vi "GFITS_writeFromBuffer.vi"(0 "total pixels":u32, 1 "log file":path, 2 "Database RefNum out":T1, 5 "bpp":i16=-32, 7 "buffer pointer":u32, 9 "name":string, 11 "error in (no error)":errorcluster) -> (15 "error out":errorcluster)   [LabVIEW 2016]
uses:
  DBSHAND/private/vis/DatabaseHand_RefNum.ctl
  DBSHAND/private/vis/DatabaseHand_Element_Set(string).vi
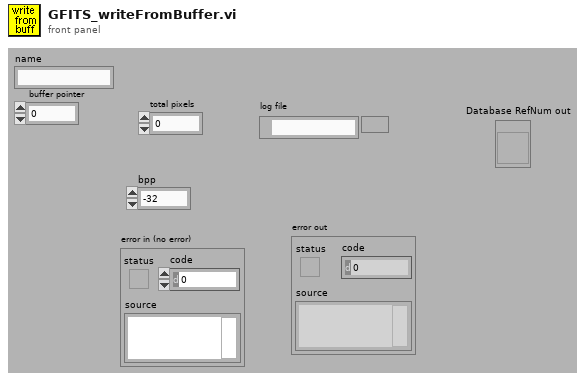
[diagram p1: front panel]
types:
  T1 = typedef "DatabaseHand_RefNum.ctl" = refnum<vi>
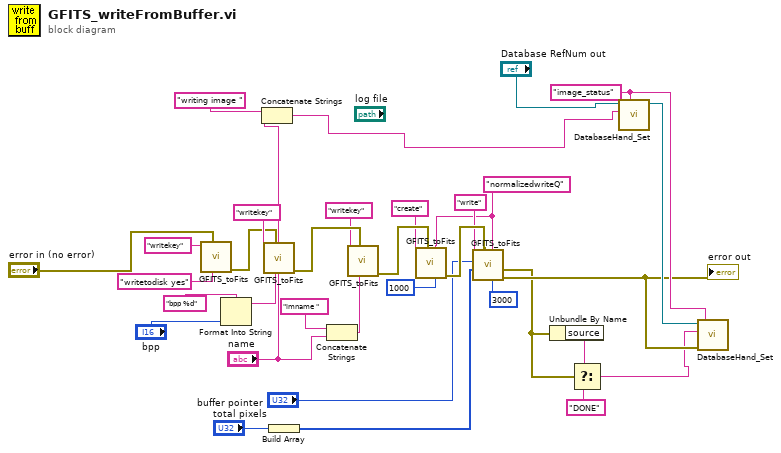
[diagram p0: block diagram]
diagram:
  w7 = "image_status" ("name")
  w13 = "normalizedwriteQ" ("response Q")
  n1 = call "GFITS_toFits.vi"("key"="writetodisk yes", "error in (no error)"="error in (no error)", "command"="writekey") -> ("error out"=w22:errorcluster)  [unwired: 6 in, 2 out]
  n2 = Format Into String(format string="bpp %d" ("Format String"), "bpp") -> (resulting string=w10:string)  [unwired: 2 in, 1 out]
  n3 = Concatenate Strings("writing image ", "name") -> (w9:string)
  n4 = call "GFITS_toFits.vi"("key"=w10, "error in (no error)"=w22, "command"="writekey") -> ("error out"=w31:errorcluster)  [unwired: 6 in, 2 out]
  n5 = Build Array("total pixels") -> (w19:u32[])
  n6 = Concatenate Strings("imname " ("key"), "name") -> (w28:string)
  n7 = call "GFITS_toFits.vi"("key"=w28, "error in (no error)"=w31, "command"="writekey") -> ("error out"=w27:errorcluster)  [unwired: 6 in, 2 out]
  n8 = call "GFITS_toFits.vi"("ms timeout (-1)"=1000, "response Q"=w13, "error in (no error)"=w27, "command"="create") -> ("error out"=w25:errorcluster)  [unwired: 5 in, 2 out]
  n9 = call "GFITS_toFits.vi"("ms timeout (-1)"=3000, "response Q"=w13, "error in (no error)"=w25, "eleRead"=w19, "location"="buffer pointer", "command"="write") -> ("error out"=w5:errorcluster, "response"=w4:errorcluster)  [unwired: 3 in, 1 out]
  "error out" <- w5
  n10 = Unbundle By Name(w4) -> ("source"=w3:string)
  n11 = Select(t=w3, s=w4, f="DONE") -> (s? t:f=w1:string)
  n12 = call-poly "DatabaseHand_Set.vi"("name"=w7, "value"=w9, "Database RefNum in"="Database RefNum out") -> ("Database RefNum out"=w6:T1)  [unwired: 5 in, 3 out]
  n13 = call-poly "DatabaseHand_Set.vi"("name"=w7, "error in (no error)"=w5, "value"=w1, "Database RefNum in"=w6) -> ()  [unwired: 4 in, 4 out]
